vi "Read Actor Queues.vi"(11 "Template in":refnum<class "Template.lvclass">) -> (3 "Base Actor Queues":T1)   [LabVIEW 2020, in "Template.lvlib" / "Template.lvclass"]
doc: "Returns the actors queues cluster"
uses:
  Template.lvclass
  typedefs/base actor queues.ctl
  Template.lvclass/Template.ctl
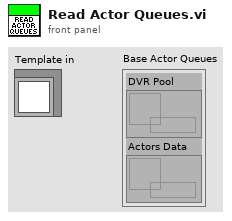
[diagram p1: front panel]
types:
  T1 = typedef "Template.lvlib/Template.lvclass/base actor queues.ctl" = cluster{"DVR Pool":refnum<queue>, "Actors Data":refnum<queue>}
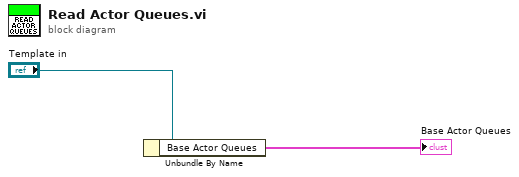
[diagram p0: block diagram]
diagram:
  n1 = Unbundle By Name("Template in") -> ("Base Actor Queues"=→"Base Actor Queues":T1)
